vi "WS1050_16 DUT VSA Save Data Ver1.3.vi"(0 "TMN DC\\CAP Data Log File Path":path=path "C:/temp", 1 "Lot#":string="WS1033", 2 "VSA_Delta C1(pF)":string[](array[string]), 4 "Wafer#":string="T4", 5 "File Name":string="Test Data", 6 "VSA_Delta C2(pF)":string[](array[string]), 7 "error in":errorcluster, 8 "Comment":string="Test Data", 9 "CP Current(uA)":string[](array[string]), 10 "VSA_IDD(A)":string="Test Data", 11 "HD Time(Min)":string="Test Data", 12 "Driver":string="Test Data", 13 "VSA_C1":string[](array[string]), 14 "CP HD (V)":string="Test Data", 15 "VSA_C2":string[](array[string]), 16 "SN":string[](array[string]), 17 "VSA_C3":string[](array[string]), 18 "Test Program":string="Test Data", 19 "Cyc_Freq(KHz)":string="Test Data", 20 "Voltage(V)":string="Test Data", 21 "Stress Voltage(V)":string="Test Data", 26 "VSA_Delta C3(pF)":string[](array[string])) -> (27 "error out":errorcluster)   [LabVIEW 2012]
panel:
  # "*********** Do Not Remove ***********\nCompany:  WiSpry Inc\n20 Fairbanks Ste 198 Irvine CA 92618\n\nAuthor:  Andy V Tran\nCreated:  09/30/2014\nLabVIEW 2012 Suite\nTP:  Multi-Socket VSA CV Save Data\n*****************************************"
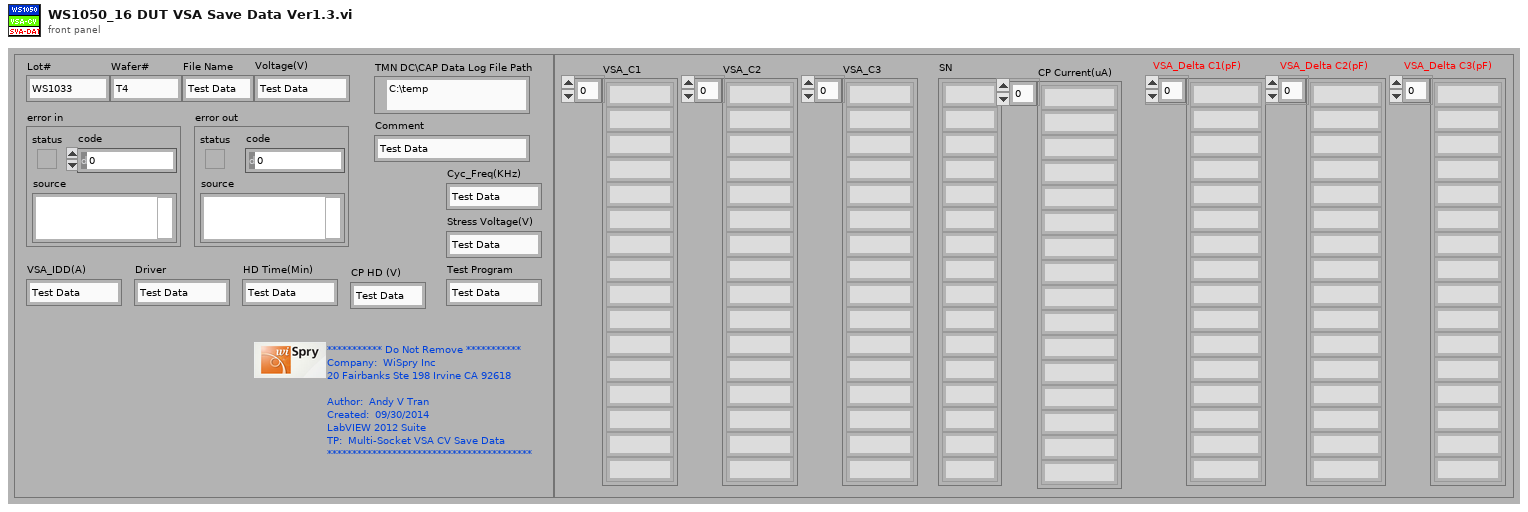
[diagram p1: front panel]
types:
  T1 = enum16{"open", "replace", "create", "open or create", "replace or create", "replace or create with confirmation"}
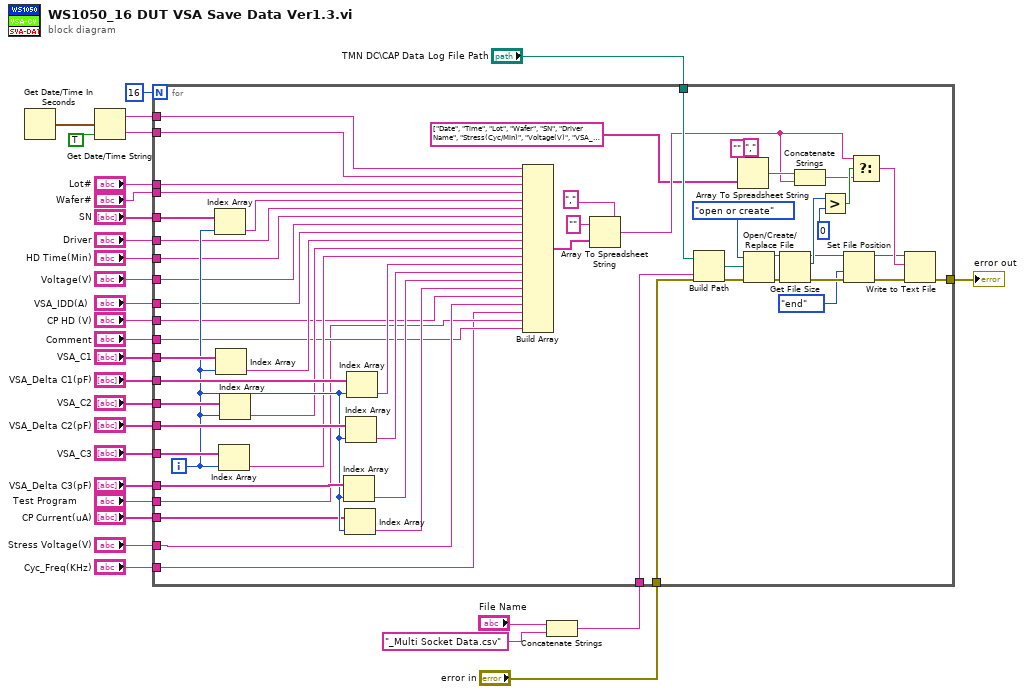
[diagram p0: block diagram]
diagram:
  n1 = Get Date/Time In Seconds() -> (seconds since 1Jan1904=w24:timestamp)
  n2 = Get Date/Time String(seconds (now)=w24, want seconds? (F)=TRUE) -> (date string=w22:string, time string=w21:string)  [unwired: 1 in]
  n3 = Concatenate Strings("File Name", "_Multi Socket Data.csv" ("string")) -> (w26:string)
  n4 = for {
    N: 16 -> [_]
    tunnel: "TMN DC\\CAP Data Log File Path" -> [w86]
    tunnel: "error in" -> [w85]
    tunnel: w26 -> [w84]
    tunnel: [w83] -> w25
    tunnel: w22 -> [w60]
    tunnel: w21 -> [w59]
    tunnel: "Lot#" -> [w58]
    tunnel: "Wafer#" -> [w57]
    tunnel: "SN" -> [w56]
    tunnel: "Voltage(V)" -> [w38]
    tunnel: "VSA_IDD(A)" -> [w39]
    tunnel: "Comment" -> [w33]
    tunnel: "VSA_C1" -> [w54]
    tunnel: "VSA_C2" -> [w53]
    tunnel: "VSA_C3" -> [w52]
    tunnel: "VSA_Delta C1(pF)" -> [w51]
    tunnel: "VSA_Delta C2(pF)" -> [w50]
    tunnel: "VSA_Delta C3(pF)" -> [w49]
    tunnel: "CP Current(uA)" -> [w47]
    tunnel: "HD Time(Min)" -> [w36]
    tunnel: "Driver" -> [w37]
    tunnel: "CP HD (V)" -> [w35]
    tunnel: "Test Program" -> [w32]
    tunnel: "Stress Voltage(V)" -> [w34]
    tunnel: "Cyc_Freq(KHz)" -> [w31]
    i -> [w48]
    n5 = Index Array(array=w56, index=w48) -> (element=w55:string)
    n6 = Index Array(array=w54, index=w48) -> (element=w40:string)
    n7 = Index Array(array=w52, index=w48) -> (element=w42:string)
    n8 = Index Array(array=w53, index=w48) -> (element=w41:string)
    n9 = Index Array(array=w49, index=w48) -> (element=w45:string)
    n10 = Index Array(array=w47, index=w48) -> (element=w46:string)
    n11 = Index Array(array=w50, index=w48) -> (element=w44:string)
    n12 = Index Array(array=w51, index=w48) -> (element=w43:string)
    n13 = Build Array(w60, w59, w58, w57, w55, w37, w36, w38, w39, w40, w41, w42, w43, w44, w45, w46, w35, w34, w31, w32, w33) -> (w61:string[])
    n14 = Array To Spreadsheet String(delimiter (Tab)=",", array=w61, 3:"" ("format string")) -> (spreadsheet string=w63:string)
    n15 = Build Path(base path=w86, name or relative path=w84) -> (appended path=w77:path)
    n16 = Array To Spreadsheet String(delimiter (Tab)=",", array=string[] ["Date", "Time", "Lot", "Wafer", "SN", "Driver Name", "Stress(Cyc/Min)", "Voltage(V)", "VSA_IDD(A)", "C1_(pF)", "C2_(pF)", "C3_(pF)", "Delta C1(pF)", "Delta C2(pF)", "Delta C3(pF)", "CP_IDD(uA)", "CP HD(V)", "Stress DCV(V)", "Cyc_Freq(KHz)", "Test Program", "Comment"], 3:"" ("format string")) -> (spreadsheet string=w65:string)
    n17 = Open/Create/Replace File(file path (use dialog)=w77, error in=w85, operation (0:open)=T1."open or create") -> (refnum out=w75:refnum<file>, error out=w78:errorcluster)  [unwired: 4 out]
    n18 = Get File Size(file=w75, error in=w78) -> (refnum out=w70:refnum<file>, size (in bytes)=w74:i64, 0:w72:errorcluster)
    n19 = Concatenate Strings(w65, w63) -> (w64:string)
    n20 = Greater?(x=w74, y=i64 0) -> (0:w79:bool)
    n21 = Set File Position(refnum=w70, from (0:start)=enum16{"start", "end", "current"}."end", error in=w72) -> (refnum out=w69:refnum<file>, error out=w71:errorcluster)  [unwired: 1 out]
    n22 = Select(t=w63, s=w79, f=w64) -> (s? t:f=w76:string)
    n23 = Write to Text File(file (use dialog)=w69, text=w76, error in=w71) -> (error out=w83:errorcluster)  [unwired: 3 out]
  }
  "error out" <- w25
